vi "VelLimiterInt32.vi"(6 "Initial Condition":i32, 9 "Limit":i32, 11 "Referenece":i32) -> (1 "coerced?":bool, 3 "VelLimitRef":i32)   [LabVIEW 2010, in "KevLib01.lvlib"]
uses:
  KevLib01.lvlib
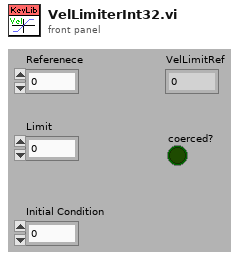
[diagram p1: front panel]
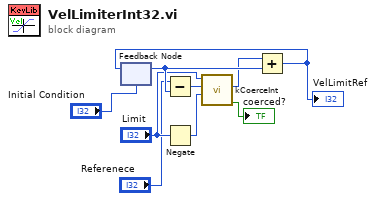
[diagram p0: block diagram]
diagram:
  n1 = feedback #1("Initial Condition") -> (w8:i32)
  n2 = Subtract(x="Referenece", y=w8) -> (x-y=w4:i32)
  n3 = Negate(x="Limit") -> (-x=w6:i32)
  n4 = call "kCoerceInt.vi"("lower"=w6, "input"=w4, "upper"="Limit") -> ("coerced?"=→"coerced?":bool, "output"=w7:i32)  [unwired: 7 out]
  n5 = Add(x=w7, y=w8) -> (x+y=w9:i32)
  "VelLimitRef" <- w9
  n6 = feedback-in #1(w9) -> ()
